vi "Update.vi"(8 "error in (no error)":errorcluster, 11 "Ramper.in":refnum<class "Ramper.lvclass">) -> (0 "error out":errorcluster, 1 "Limit Reached":bool, 2 "Incremented":bool, 3 "Ramper.out":refnum<class "Ramper.lvclass">)   [LabVIEW 2014, in "Ramper.lvclass"]
uses:
  Ramper.lvclass
  Ramper.lvclass/Ramper.ctl
  <vilib>/gmath/NI_Gmath.lvlib
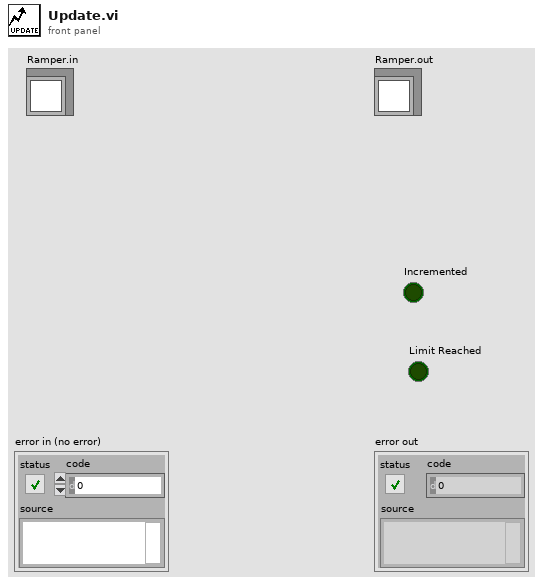
[diagram p1: front panel]
types:
  T1 = cluster{"Y Values":dbl[][], "Tables":i32[][][], "Variables input decode":i32[], "Variables output decode":i32[]}
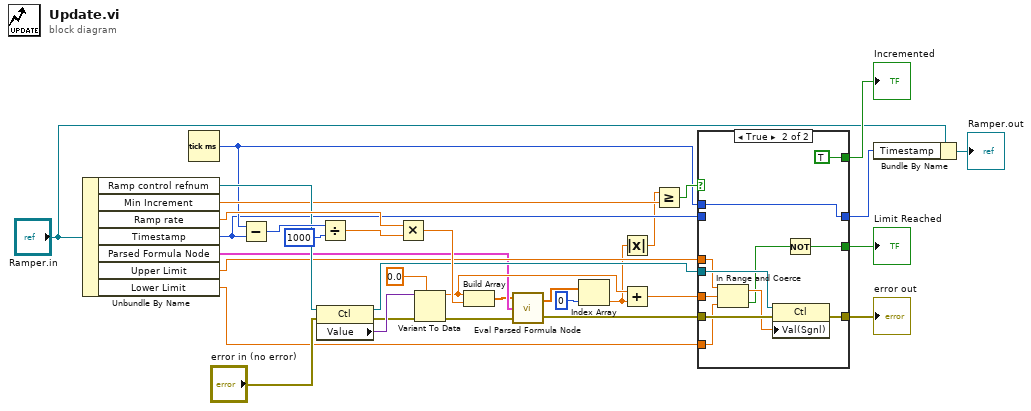
[diagram p0: block diagram]
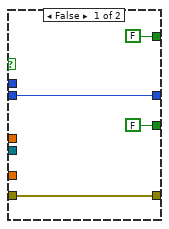
[diagram p2: hidden frame]
diagram:
  n1 = Unbundle By Name("Ramper.in") -> ("Ramp control refnum"=w29:refnum<vi>, "Min Increment"=w23:dbl, "Ramp rate"=w30:dbl, "Timestamp"=w15:u32, "Parsed Formula Node"=w7:T1, "Upper Limit"=w9:dbl, "Lower Limit"=w8:dbl)
  n2 = Tick Count (ms)() -> (millisecond timer value=w17:u32)
  n3 = Subtract(x=w17, y=w15) -> (x-y=w33:u32)
  n4 = property class="Ctl"(reference=w29, error in="error in (no error)") -> (reference out=w16:refnum<vi>, error out=w25:errorcluster, "Value"=w27:variant)
  n5 = Divide(x=w33, y=u32 1000) -> (x/y=w31:dbl)
  n6 = Multiply(x=w30, y=w31) -> (x*y=w24:dbl)
  n7 = Variant To Data(error in=w25, type=0.0, Variant=w27) -> (data=w13:dbl, error out=w5:errorcluster)
  n8 = Build Array(w13, w24) -> (w6:dbl[])
  n9 = call <vilib>:"Eval Parsed Formula Node.vi"("error in (no error)"=w5, "Parsed Formula Node"=w7, "Input Values"=w6) -> ("error out"=w4:errorcluster, "Output Values"=w3:dbl[])
  n10 = Index Array(array=w3, index=0) -> (element=w1:dbl)
  n11 = Absolute Value(x=w1) -> (abs(x)=w11:dbl)
  n12 = Add(x=w13, y=w1) -> (x+y=w12:dbl)
  n13 = Greater Or Equal?(x=w11, y=w23) -> (x >= y?=w21:bool)
  n14 = case shown="True" w21 {
    tunnel: [FALSE TRUE] -> w22
    tunnel: [w37 w48] -> w18
    tunnel: w17 -> [_ w48]
    tunnel: w4 -> [w36 w46]
    tunnel: w16 -> [_ w47]
    tunnel: [w36 w45] -> w14
    tunnel: w15 -> [w37 _]
    tunnel: w12 -> [_ w41]
    tunnel: [FALSE w39] -> w10
    tunnel: w9 -> [_ w43]
    tunnel: w8 -> [_ w42]
    frame False {
    }
    frame True {
      n15 = In Range and Coerce(upper limit=w43, x=w41, lower limit=w42) -> (coerced(x)=w40:dbl, In Range?=w38:bool)
      n16 = property class="Ctl"(reference=w47, error in=w46, "Val(Sgnl)"=w40) -> (error out=w45:errorcluster)  [unwired: 1 out]
      n17 = Not(x=w38) -> (.not. x?=w39:bool)
    }
  }
  "error out" <- w14
  "Incremented" <- w22
  "Limit Reached" <- w10
  n18 = Bundle By Name(cluster="Ramper.in", "Timestamp"=w18) -> (→"Ramper.out":refnum<class "Ramper.lvclass">)
